vi "_Serial FPGA Send.vi"(0 "LED Control (T)":bool=TRUE) -> ()   [LabVIEW 2012]
uses:
  <vilib>/rvi/Emulation/niFpgaSctlEmulationGetInTimedLoop.vi
  <vilib>/rvi/Emulation/niFpgaSctlEmulationGlobalWrite.vi
  <vilib>/rvi/Memory/Memory_Emulation/nirvimemoryEmulationManagerCache_ReleaseExclusive.vi
  <vilib>/rvi/Memory/Memory_Emulation/niFpgaMemoryEmulationValidateCache.vi
  <vilib>/rvi/Memory/Memory_Emulation/nirvimemoryEmulationManagerCache_MakeExclusive.vi
  <vilib>/rvi/Memory/Memory_Emulation/niFpgaMemoryEmulationCacheClearOnFirstRun.vi
  <vilib>/rvi/DataTransferAndStorage/Container/Common/niFpgaContainerGetUniqueNameForEmu.vi
  <vilib>/rvi/Memory/Memory_Emulation/nirvimemoryEmulationManagerCache_InsertValue.vi
  <vilib>/Utility/error.llb/Clear Errors.vi
  <vilib>/rvi/Memory/Memory_Emulation/nirvimemoryEmulationManagerCache_SetValue.vi
  <vilib>/rvi/Memory/Memory_Emulation/nirvimemoryEmulationManagerCache_GetValue.vi
  <vilib>/rvi/Emulation/niFpgaSctlEmulationResourceMgr.vi
  <vilib>/rvi/eio/common/nirviEmuTemplateMethod_errors.vi
  <vilib>/rvi/DataTransferAndStorage/Container/XNode/niFpgaContainer.xnode
  <vilib>/rvi/Memory/Memory_Emulation/nirvimemoryEmulation.vi
  <vilib>/eio/EIONode/EIONode.xnode
  <vilib>/eio/EIOMethodNode/EIOMethodNode.xnode
panel:
  out "Bytes Written":u8
  out "Bytes Read":u8
  out "Done":bool
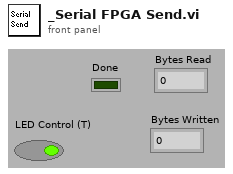
[diagram p1: front panel]
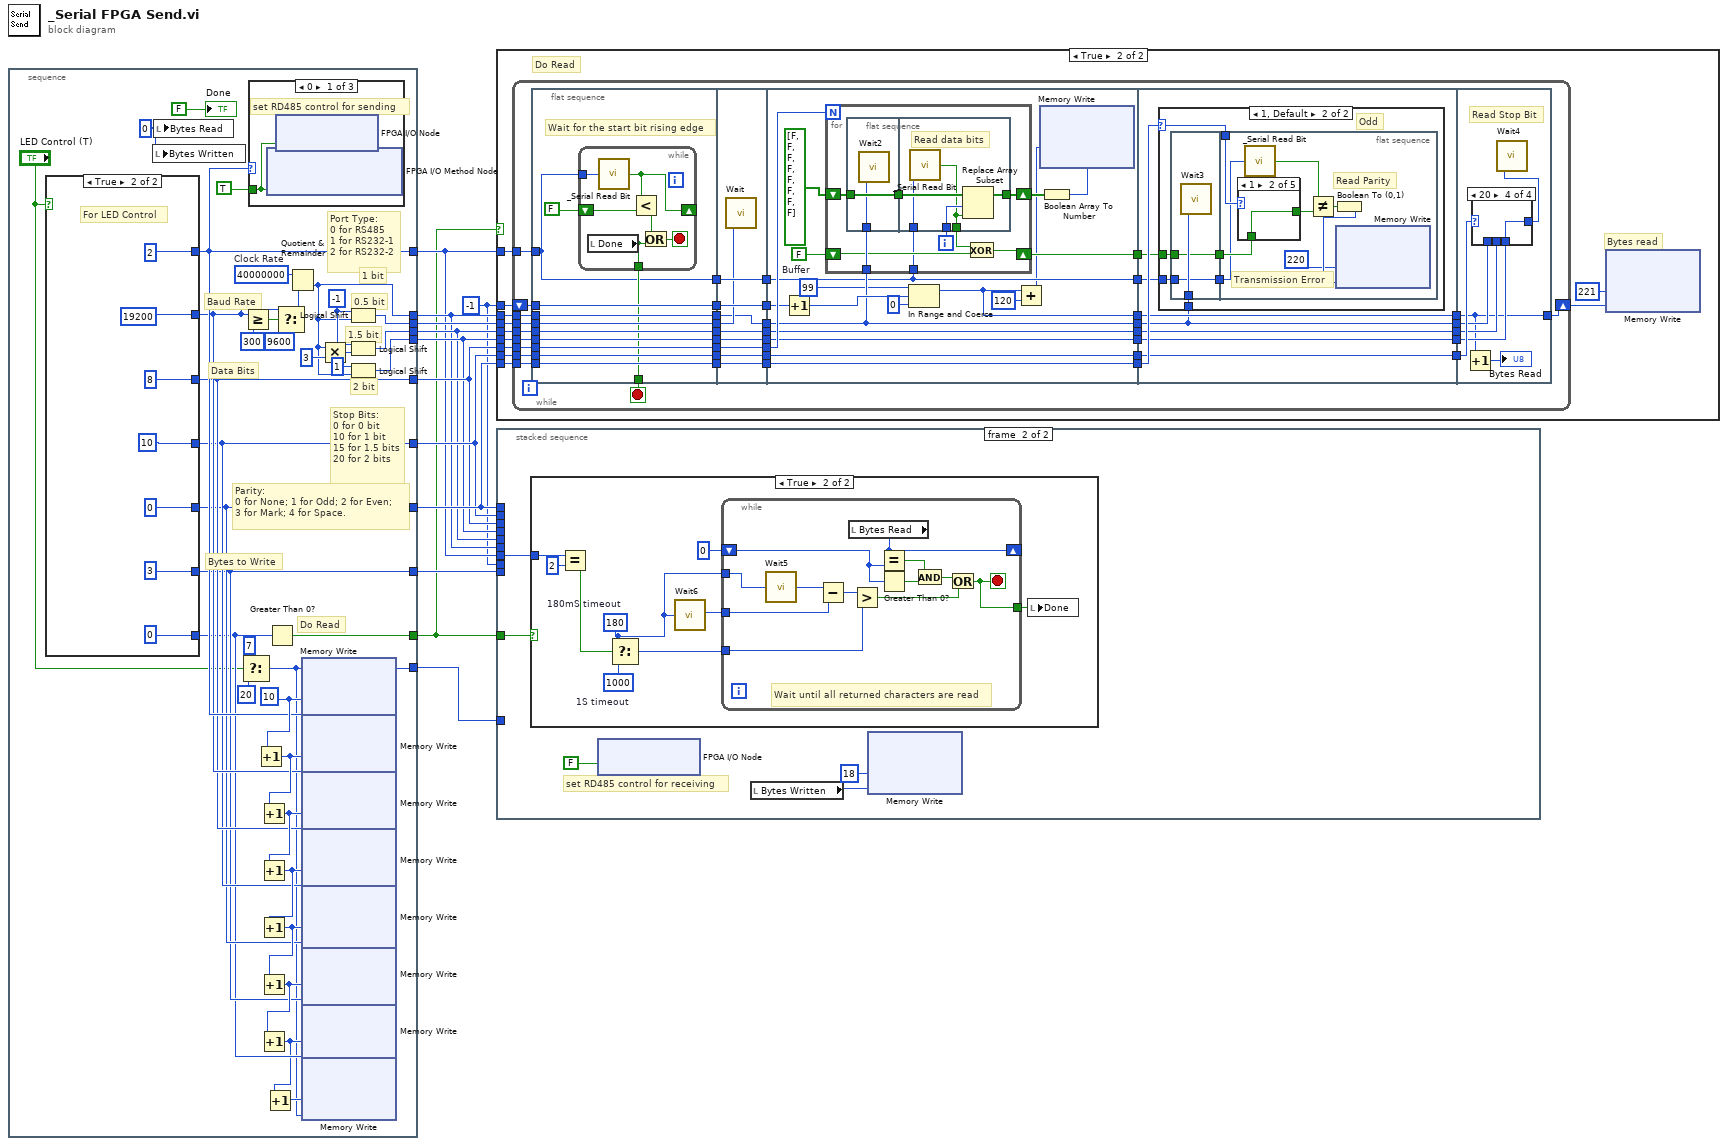
[diagram p0: block diagram]
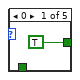
[diagram p4: hidden frame]
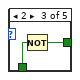
[diagram p5: hidden frame]
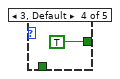
[diagram p6: hidden frame]
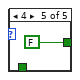
[diagram p7: hidden frame]
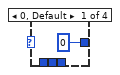
[diagram p8: hidden frame]
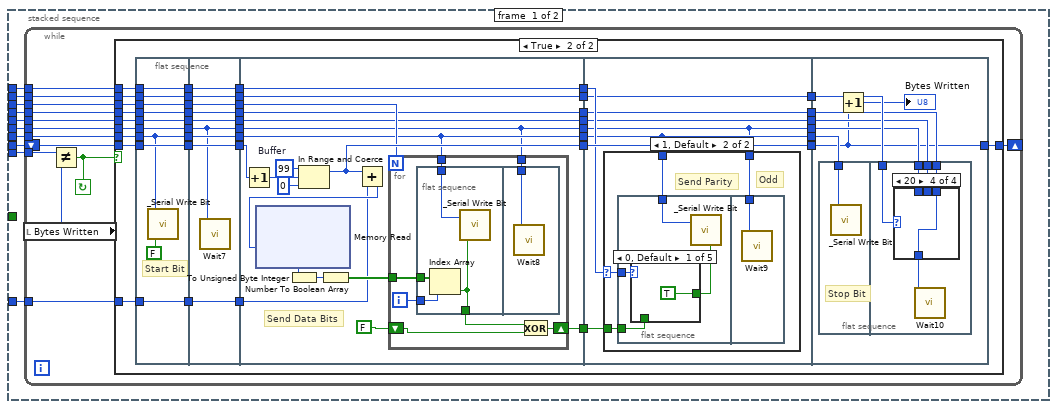
[diagram p11: hidden frame]
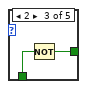
[diagram p15: hidden frame]
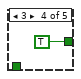
[diagram p16: hidden frame]
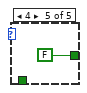
[diagram p17: hidden frame]
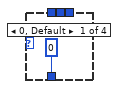
[diagram p18: hidden frame]
diagram:
  w3 = i16 -1
  n1 = stacked-sequence {
    tunnel: [w37] -> w5
    tunnel: [w40] -> w12
    tunnel: [w39] -> w6
    tunnel: [w36] -> w7
    tunnel: [w22] -> w8
    tunnel: [w24] -> w4
    tunnel: [w21] -> w9
    tunnel: [w20] -> w10
    tunnel: [w19] -> w11
    tunnel: [w32] -> w2
    tunnel: [w15] -> w1
    frame #0 {
      w29 = u8 10 ("Address")
      w42 = i16 -1 ("y")
      w44 = u32 40000000  # Clock Rate
      w34 = u8 0 ("Bytes Read")
      # "Do Read"
      # "1.5 bit"
      # "2 bit"
      # "0.5 bit"
      # "1 bit"
      # "Bytes to Write"
      # "Parity:\n0 for None; 1 for Odd; 2 for Even;\n3 for Mark; 4 for Space."
      # "Stop Bits:\n0 for 0 bit\n10 for 1 bit\n15 for 1.5 bits\n20 for 2 bits"
      # "Data Bits"
      # "Baud Rate"
      # "Port Type: \n0 for RS485\n1 for RS232-1\n2 for RS232-2"
      n2 = case shown="True" "LED Control (T)" {
        tunnel: [w57 u8 8 ("Address")] -> w22
        tunnel: [w56 u8 10 ("Address")] -> w21
        tunnel: [w55 u8 0 ("Address")] -> w20
        tunnel: [w54 u8 3 ("Address")] -> w19
        tunnel: [w53 u16 19200 ("Address")] -> w23
        tunnel: [w52 u8 2 ("Address")] -> w24
        tunnel: [w49 u8 0 ("Address")] -> w18
        frame False {
          w62 = u8 0 ("Address")
          n3 = Increment(x=w62) -> (x+1=w61:u8)
          n4 = Increment(x=w61) -> (x+1=w60:u8)
          n5 = Increment(x=w60) -> (x+1=w59:u8)
          n6 = Increment(x=w59) -> (x+1=w58:u8)
          n7 = Increment(x=w58) -> (x+1=w50:u8)
          n8 = Increment(x=w50) -> (x+1=w51:u8)
          n9 = xnode ("Memory Read")("Address"=w62) -> ("Data"=w52:u32)  [unwired: 1 in, 1 out]
          n10 = xnode ("Memory Read")("Address"=w61) -> ("Data"=w53:u32)  [unwired: 1 in, 1 out]
          n11 = xnode ("Memory Read")("Address"=w60) -> ("Data"=w57:u32)  [unwired: 1 in, 1 out]
          n12 = xnode ("Memory Read")("Address"=w59) -> ("Data"=w56:u32)  [unwired: 1 in, 1 out]
          n13 = xnode ("Memory Read")("Address"=w58) -> ("Data"=w55:u32)  [unwired: 1 in, 1 out]
          n14 = xnode ("Memory Read")("Address"=w50) -> ("Data"=w54:u32)  [unwired: 1 in, 1 out]
          n15 = xnode ("Memory Read")("Address"=w51) -> ("Data"=w49:u32)  [unwired: 1 in, 1 out]
        }
        frame True {
          # "For LED Control"
        }
      }
      n16 = local write "Bytes Written"(w34) -> ()
      n17 = local write "Bytes Read"(w34) -> ()
      n18 = Select(t=u8 7 ("y"), s="LED Control (T)", f=u8 20 ("y")) -> (s? t:f=w15:u8)
      n19 = Greater Or Equal?(x=w23, y=u16 300) -> (x >= y?=w47:bool)
      n20 = case shown="0" w24 {
        tunnel: TRUE -> [w70 w71 w72]
        frame 0 {
          # "set RD485 control for sending"
          n21 = xnode "FPGA I/O Method Node"("Enable"=w70) -> ()  [unwired: 1 in, 1 out]
          n22 = xnode "FPGA I/O Node"("Port5/DIO4"=w70) -> ()  [unwired: 1 in, 1 out]
        }
        frame 1, Default {
          n23 = xnode "FPGA I/O Method Node"("Enable"=w71) -> ()  [unwired: 1 in, 1 out]
        }
        frame 2 {
          # "LCD/LED Control"
          n24 = xnode "FPGA I/O Method Node"("Enable"=w72) -> ()  [unwired: 1 in, 1 out]
        }
      }
      n25 = Increment(x=w29) -> (x+1=w30:u8)
      n26 = Increment(x=w30) -> (x+1=w28:u8)
      n27 = Increment(x=w28) -> (x+1=w27:u8)
      n28 = Increment(x=w27) -> (x+1=w26:u8)
      n29 = Increment(x=w26) -> (x+1=w25:u8)
      n30 = Increment(x=w25) -> (x+1=w16:u8)
      n31 = Increment(x=w16) -> (x+1=w17:u8)
      n32 = Greater Than 0?(x=w18) -> (x > 0?=w32:bool)
      n33 = Select(t=w23, s=w47, f=u16 9600) -> (s? t:f=w45:u32)
      n34 = Quotient & Remainder(x=w44, y=w45) -> (floor(x/y)=w37:u32)  [unwired: 1 out]
      n35 = xnode ("Memory Write")("Address"=w29, "Data"=w24) -> ()  [unwired: 1 in, 1 out]
      n36 = xnode ("Memory Write")("Address"=w30, "Data"=w23) -> ()  [unwired: 1 in, 1 out]
      n37 = xnode ("Memory Write")("Address"=w28, "Data"=w22) -> ()  [unwired: 1 in, 1 out]
      n38 = xnode ("Memory Write")("Address"=w27, "Data"=w21) -> ()  [unwired: 1 in, 1 out]
      n39 = xnode ("Memory Write")("Address"=w26, "Data"=w20) -> ()  [unwired: 1 in, 1 out]
      n40 = xnode ("Memory Write")("Address"=w25, "Data"=w19) -> ()  [unwired: 1 in, 1 out]
      n41 = xnode ("Memory Write")("Address"=w16, "Data"=w18) -> ()  [unwired: 1 in, 1 out]
      n42 = xnode ("Memory Write")("Address"=w17, "Data"=w15) -> ()  [unwired: 1 in, 1 out]
      n43 = Multiply(x=w37, y=u32 3) -> (x*y=w41:u32)
      n44 = Logical Shift(y=w42, x=w37) -> (x << y=w40:u32)
      n45 = Logical Shift(y=w42, x=w41) -> (x << y=w39:u32)
      n46 = Logical Shift(y=i16 1, x=w37) -> (x << y=w36:u32)
      "Done" <- FALSE ("Done")
    }
  }
  n47 = case shown="True" w2 {
    tunnel: w12 -> [_ w83]
    tunnel: w10 -> [_ w82]
    tunnel: w9 -> [_ w81]
    tunnel: w8 -> [_ w80]
    tunnel: w7 -> [_ w79]
    tunnel: w6 -> [_ w78]
    tunnel: w5 -> [_ w77]
    tunnel: w4 -> [_ w76]
    tunnel: w3 -> [_ w75]
    frame False {
    }
    frame True {
      # "Bytes read"
      # "Do Read"
      n48 = while {
        tunnel: w79 -> [w121]
        tunnel: w78 -> [w122]
        tunnel: w83 -> [w123]
        tunnel: w77 -> [w124]
        tunnel: w76 -> [w104]
        shift-right: [w84] -> w73
        shift-left: w75 -> [w102]
        tunnel: w80 -> [w120]
        tunnel: w81 -> [w119]
        tunnel: w82 -> [w118]
        stop <- w85 stop-if-true
        n49 = flat-sequence {
          tunnel: w118 -> [w129]
          tunnel: w119 -> [w130]
          tunnel: w120 -> [w131]
          tunnel: w121 -> [w132]
          tunnel: w122 -> [w133]
          tunnel: w123 -> [w134]
          tunnel: w124 -> [w135]
          tunnel: [w135] -> w111
          tunnel: [w134] -> w110
          tunnel: [w133] -> w109
          tunnel: [w132] -> w108
          tunnel: [w131] -> w107
          tunnel: [w130] -> w106
          tunnel: [w129] -> w105
          tunnel: w104 -> [w125]
          tunnel: [w128] -> w103
          tunnel: w102 -> [w128]
          tunnel: [w125] -> w99
          tunnel: [w126] -> w85
          tunnel: [w142] -> w117
          tunnel: [w150] -> w116
          tunnel: [w149] -> w115
          tunnel: [w148] -> w114
          tunnel: [w147] -> w113
          tunnel: [w146] -> w112
          tunnel: w111 -> [w142]
          tunnel: w110 -> [w143]
          tunnel: w109 -> [w150]
          tunnel: w108 -> [w149]
          tunnel: w107 -> [w148]
          tunnel: w106 -> [w147]
          tunnel: w105 -> [w146]
          tunnel: w103 -> [w145]
          tunnel: [w145] -> w101
          tunnel: [w144] -> w100
          tunnel: w99 -> [w144]
          tunnel: w117 -> [w159]
          tunnel: w116 -> [w156]
          tunnel: w115 -> [w155]
          tunnel: w114 -> [w167]
          tunnel: w113 -> [w157]
          tunnel: w112 -> [w160]
          tunnel: w101 -> [w166]
          tunnel: w100 -> [w154]
          tunnel: [w161] -> w98
          tunnel: [w160] -> w97
          tunnel: [w159] -> w96
          tunnel: [w154] -> w95
          tunnel: [w158] -> w94
          tunnel: [w157] -> w91
          tunnel: [w156] -> w88
          tunnel: [w155] -> w86
          tunnel: w98 -> [w192]
          tunnel: w97 -> [w193]
          tunnel: w96 -> [w188]
          tunnel: w95 -> [w191]
          tunnel: w94 -> [w190]
          tunnel: [w190] -> w93
          tunnel: [w189] -> w92
          tunnel: w91 -> [w189]
          tunnel: [w188] -> w90
          tunnel: [w187] -> w89
          tunnel: w88 -> [w187]
          tunnel: [w186] -> w87
          tunnel: w86 -> [w186]
          tunnel: w93 -> [w218]
          tunnel: w92 -> [w223]
          tunnel: w90 -> [w221]
          tunnel: w89 -> [w220]
          tunnel: w87 -> [w219]
          tunnel: [w218] -> w84
          frame #0 {
            # "Wait for the start bit rising edge"
            n50 = while {
              shift-right: [w137] -> _
              shift-left: FALSE -> [w141]
              tunnel: w125 -> [w140]
              tunnel: [w136] -> w126
              stop <- w138 stop-if-true
              n51 = local read "Done"() -> (w136:bool)
              n52 = call "_Serial Read Bit.vi"("Port type"=w140) -> ("BitState"=w137:bool)
              n53 = Less?(x=w137, y=w141) -> (x < y?=w139:bool)
              n54 = Or(x=w139, y=w136) -> (x .or. y?=w138:bool)
            }
          }
          frame #1 {
            n55 = call "Wait"("Count(Ticks)"=w143) -> ()  [unwired: 1 out]
          }
          frame #2 {
            w152 = i16 99  # Buffer
            n56 = Increment(x=w166) -> (x+1=w165:i16)
            n57 = for {
              N: w167 -> [_]
              shift-right: [w172] -> w162
              shift-left: bool[] [FALSE, FALSE, FALSE, FALSE, FALSE, FALSE, FALSE, FALSE] -> [w178]
              tunnel: w159 -> [w176]
              shift-right: [w175] -> w161
              shift-left: FALSE -> [w174]
              tunnel: w154 -> [w170]
              i -> [w171]
              n58 = flat-sequence {
                tunnel: w178 -> [w180]
                tunnel: [w180] -> w177
                tunnel: w176 -> [w179]
                tunnel: w171 -> [w185]
                tunnel: w177 -> [w184]
                tunnel: [w183] -> w172
                tunnel: [w181] -> w173
                tunnel: w170 -> [w182]
                frame #0 {
                  n59 = call "Wait2"("Count(Ticks)"=w179) -> ()  [unwired: 1 out]
                }
                frame #1 {
                  # "Read data bits"
                  n60 = call "_Serial Read Bit.vi"("Port type"=w182) -> ("BitState"=w181:bool)
                  n61 = Replace Array Subset(array=w184, new element=w181, index=w185) -> (w183:bool[])
                }
              }
              n62 = Exclusive Or(1:w174, 2:w173) -> (0:w175:bool)
            }
            n63 = In Range and Coerce(upper limit=w152, x=w165, lower limit=i16 0) -> (coerced(x)=w158:i16)  [unwired: 1 out]
            n64 = Add(x=w158, y=i16 120) -> (x+y=w153:i16)
            n65 = Boolean Array To Number(Boolean array=w162) -> (number=w151:u8)
            n66 = xnode ("Memory Write")("Address"=w153, "Data"=w151) -> ()  [unwired: 1 in, 1 out]
          }
          frame #3 {
            n67 = case shown="1, Default" w193 {
              selector: w193 -> [_ w198]
              tunnel: w192 -> [_ w196]
              tunnel: w188 -> [_ w199]
              tunnel: w191 -> [_ w194]
              frame 0 {
                # "None"
              }
              frame 1, Default {
                # "Odd"
                n68 = flat-sequence {
                  tunnel: w199 -> [w202]
                  tunnel: [w201] -> w197
                  tunnel: w196 -> [w201]
                  tunnel: [w200] -> w195
                  tunnel: w194 -> [w200]
                  tunnel: w198 -> [w210]
                  tunnel: w197 -> [w208]
                  tunnel: w195 -> [w204]
                  frame #0 {
                    n69 = call "Wait3"("Count(Ticks)"=w202) -> ()  [unwired: 1 out]
                  }
                  frame #1 {
                    # "Read Parity"
                    # "Transmission Error"
                    n70 = case shown="1" w210 {
                      tunnel: w208 -> [_ w212 w214 _ _]
                      tunnel: [TRUE ("y") w212 w213 TRUE ("y") FALSE ("y")] -> w209
                      frame 0 {
                      }
                      frame 1 {
                      }
                      frame 2 {
                        n71 = Not(x=w214) -> (.not. x?=w213:bool)
                      }
                      frame 3, Default {
                      }
                      frame 4 {
                      }
                    }
                    n72 = call "_Serial Read Bit.vi"("Port type"=w204) -> ("BitState"=w203:bool)
                    n73 = Not Equal?(x=w203, y=w209) -> (x != y?=w207:bool)
                    n74 = Boolean To (0,1)(Boolean=w207) -> (0, 1=w206:i16)
                    n75 = xnode ("Memory Write")("Address"=u16 220 ("y"), "Data"=w206) -> ()  [unwired: 1 in, 1 out]
                  }
                }
              }
            }
          }
          frame #4 {
            # "Read Stop Bit"
            n76 = Increment(x=w218) -> (x+1=→"Bytes Read":i16)
            n77 = case shown="20" w223 {
              tunnel: w221 -> [_ w225 _ _]
              tunnel: w220 -> [_ _ w226 _]
              tunnel: w219 -> [_ _ _ w227]
              tunnel: [u32 0 ("One Bit") w225 w226 w227] -> w222
              frame 0, Default {
              }
              frame 10 {
              }
              frame 15 {
              }
              frame 20 {
              }
            }
            n78 = call "Wait4"("Count(Ticks)"=w222) -> ()  [unwired: 1 out]
          }
        }
      }
      n79 = xnode ("Memory Write")("Address"=u16 221 ("y"), "Data"=w73) -> ()  [unwired: 1 in, 1 out]
    }
  }
  n80 = stacked-sequence {
    tunnel: w11 -> [w237 _]
    tunnel: w10 -> [w236 _]
    tunnel: w9 -> [w235 _]
    tunnel: w8 -> [w234 _]
    tunnel: w7 -> [w233 _]
    tunnel: w6 -> [w232 _]
    tunnel: w5 -> [w231 _]
    tunnel: w4 -> [w230 w384]
    tunnel: w3 -> [w229 _]
    tunnel: w2 -> [_ w387]
    tunnel: w1 -> [w228 _]
    frame #0 {
      n81 = while {
        tunnel: w237 -> [w250]
        tunnel: w236 -> [w247]
        tunnel: w235 -> [w246]
        tunnel: w234 -> [w245]
        tunnel: w233 -> [w244]
        tunnel: w232 -> [w243]
        tunnel: w231 -> [w242]
        tunnel: w230 -> [w241]
        shift-right: [w239] -> _
        shift-left: w229 -> [w240]
        tunnel: w228 -> [w238]
        stop <- w248 continue-if-true
        n82 = local read "Bytes Written"() -> (w249:u8)
        n83 = Not Equal?(x=w250, y=w249) -> (x != y?=w248:bool)
        n84 = case shown="True" w248 {
          tunnel: w247 -> [_ w275]
          tunnel: w246 -> [_ w266]
          tunnel: w245 -> [_ w284]
          tunnel: w244 -> [_ w255]
          tunnel: w243 -> [_ w260]
          tunnel: w242 -> [_ w289]
          tunnel: w241 -> [_ w293]
          tunnel: w240 -> [w251 w291]
          tunnel: [w251 w287] -> w239
          tunnel: w238 -> [_ w252]
          frame False {
          }
          frame True {
            n85 = flat-sequence {
              tunnel: w293 -> [w300]
              tunnel: [w303] -> w292
              tunnel: w291 -> [w303]
              tunnel: [w302] -> w290
              tunnel: w289 -> [w302]
              tunnel: [w301] -> w285
              tunnel: w284 -> [w301]
              tunnel: [w300] -> w282
              tunnel: [w299] -> w276
              tunnel: w275 -> [w299]
              tunnel: [w298] -> w267
              tunnel: w266 -> [w298]
              tunnel: [w297] -> w261
              tunnel: w260 -> [w297]
              tunnel: [w296] -> w256
              tunnel: w255 -> [w296]
              tunnel: [w294] -> w253
              tunnel: w252 -> [w294]
              tunnel: w292 -> [w312]
              tunnel: w290 -> [w309]
              tunnel: [w312] -> w288
              tunnel: [w311] -> w286
              tunnel: w285 -> [w311]
              tunnel: [w310] -> w283
              tunnel: w282 -> [w310]
              tunnel: [w309] -> w281
              tunnel: [w308] -> w277
              tunnel: w276 -> [w308]
              tunnel: [w307] -> w268
              tunnel: w267 -> [w307]
              tunnel: [w306] -> w262
              tunnel: w261 -> [w306]
              tunnel: [w305] -> w257
              tunnel: w256 -> [w305]
              tunnel: [w304] -> w254
              tunnel: w253 -> [w304]
              tunnel: w288 -> [w331]
              tunnel: w286 -> [w323]
              tunnel: w283 -> [w318]
              tunnel: w281 -> [w317]
              tunnel: [w324] -> w280
              tunnel: [w320] -> w279
              tunnel: [w319] -> w278
              tunnel: w277 -> [w319]
              tunnel: [w318] -> w274
              tunnel: [w317] -> w273
              tunnel: [w316] -> w269
              tunnel: w268 -> [w316]
              tunnel: [w315] -> w263
              tunnel: w262 -> [w315]
              tunnel: [w314] -> w258
              tunnel: w257 -> [w314]
              tunnel: w254 -> [w313]
              tunnel: w280 -> [w351]
              tunnel: w279 -> [w349]
              tunnel: w278 -> [w350]
              tunnel: w274 -> [w348]
              tunnel: w273 -> [w346]
              tunnel: [w351] -> w272
              tunnel: [w348] -> w271
              tunnel: [w347] -> w270
              tunnel: w269 -> [w347]
              tunnel: [w346] -> w265
              tunnel: [w345] -> w264
              tunnel: w263 -> [w345]
              tunnel: [w344] -> w259
              tunnel: w258 -> [w344]
              tunnel: [w368] -> w287
              tunnel: w272 -> [w368]
              tunnel: w271 -> [w373]
              tunnel: w270 -> [w372]
              tunnel: w265 -> [w371]
              tunnel: w264 -> [w370]
              tunnel: w259 -> [w369]
              frame #0 {
                # "Start Bit"
                n86 = call "_Serial Write Bit.vi"("BitState(T)"=FALSE, "Port type"=w300) -> ()  [unwired: 1 out]
              }
              frame #1 {
                n87 = call "Wait7"("Count(Ticks)"=w309) -> ()  [unwired: 1 out]
              }
              frame #2 {
                w329 = i16 99  # Buffer
                # "Send Data Bits"
                n88 = Increment(x=w331) -> (x+1=w330:i16)
                n89 = In Range and Coerce(upper limit=w329, x=w330, lower limit=i16 0) -> (coerced(x)=w324:i16)  [unwired: 1 out]
                n90 = Add(x=w324, y=w313) -> (x+y=w327:i16)
                n91 = xnode ("Memory Read")("Address"=w327) -> ("Data"=w325:u32)  [unwired: 1 in, 1 out]
                n92 = To Unsigned Byte Integer(number=w325) -> (unsigned 8bit integer=w326:u8)
                n93 = Number To Boolean Array(number=w326) -> (Boolean array=w322:bool[])
                n94 = for {
                  N: w323 -> [_]
                  tunnel: w322 -> [w338]
                  shift-right: [w336] -> w320
                  shift-left: FALSE -> [w335]
                  tunnel: w318 -> [w333]
                  tunnel: w317 -> [w332]
                  i -> [w337]
                  n95 = flat-sequence {
                    tunnel: w338 -> [w342]
                    tunnel: w337 -> [w341]
                    tunnel: [w339] -> w334
                    tunnel: w333 -> [w340]
                    tunnel: w332 -> [w343]
                    frame #0 {
                      n96 = Index Array(array=w342, index=w341) -> (element=w339:bool)
                      n97 = call "_Serial Write Bit.vi"("BitState(T)"=w339, "Port type"=w340) -> ()  [unwired: 1 out]
                    }
                    frame #1 {
                      n98 = call "Wait8"("Count(Ticks)"=w343) -> ()  [unwired: 1 out]
                    }
                  }
                  n99 = Exclusive Or(1:w335, 2:w334) -> (0:w336:bool)
                }
              }
              frame #3 {
                n100 = case shown="1, Default" w350 {
                  selector: w350 -> [_ w355]
                  tunnel: w349 -> [_ w354]
                  tunnel: w348 -> [_ w353]
                  tunnel: w346 -> [_ w352]
                  frame 0 {
                    # "None"
                  }
                  frame 1, Default {
                    # "Send Parity"
                    # "Odd"
                    n101 = flat-sequence {
                      tunnel: w355 -> [w359]
                      tunnel: w354 -> [w358]
                      tunnel: w353 -> [w356]
                      tunnel: w352 -> [w366]
                      frame #0 {
                        n102 = case shown="0, Default" w359 {
                          tunnel: w358 -> [_ w361 w363 _ _]
                          tunnel: [TRUE ("y") w361 w362 TRUE ("y") FALSE ("y")] -> w357
                          frame 0, Default {
                          }
                          frame 1 {
                          }
                          frame 2 {
                            n103 = Not(x=w363) -> (.not. x?=w362:bool)
                          }
                          frame 3 {
                          }
                          frame 4 {
                          }
                        }
                        n104 = call "_Serial Write Bit.vi"("BitState(T)"=w357, "Port type"=w356) -> ()  [unwired: 1 out]
                      }
                      frame #1 {
                        n105 = call "Wait9"("Count(Ticks)"=w366) -> ()  [unwired: 1 out]
                      }
                    }
                  }
                }
              }
              frame #4 {
                n106 = flat-sequence {
                  tunnel: w373 -> [w374]
                  tunnel: w372 -> [w379]
                  tunnel: w371 -> [w377]
                  tunnel: w370 -> [w376]
                  tunnel: w369 -> [w375]
                  frame #0 {
                    # "Stop Bit"
                    n107 = call "_Serial Write Bit.vi"("Port type"=w374) -> ()  [unwired: 1 in, 1 out]
                  }
                  frame #1 {
                    n108 = case shown="20" w379 {
                      tunnel: [u32 0 ("One Bit") w381 w382 w383] -> w378
                      tunnel: w377 -> [_ w381 _ _]
                      tunnel: w376 -> [_ _ w382 _]
                      tunnel: w375 -> [_ _ _ w383]
                      frame 0, Default {
                      }
                      frame 10 {
                      }
                      frame 15 {
                      }
                      frame 20 {
                      }
                    }
                    n109 = call "Wait10"("Count(Ticks)"=w378) -> ()  [unwired: 1 out]
                  }
                }
                n110 = Increment(x=w368) -> (x+1=→"Bytes Written":i16)
              }
            }
          }
        }
      }
    }
    frame #1 {
      # "set RD485 control for receiving"
      n111 = case shown="True" w387 {
        tunnel: w384 -> [_ w394]
        frame False {
        }
        frame True {
          w389 = u32 180  # 180mS timeout
          w391 = u32 1000  # 1S timeout
          n112 = Equal?(x=w394, y=u32 2) -> (x = y?=w392:bool)
          n113 = Select(t=w389, s=w392, f=w391) -> (s? t:f=w390:u32)
          n114 = call "Wait6"("Count(mSec)"=w389) -> ("Tick Count(mSec)"=w395:u32)
          n115 = while {
            tunnel: w395 -> [w408]
            shift-right: [w406] -> _
            shift-left: u8 0 ("Bytes Read") -> [w405]
            tunnel: [w400] -> w396
            tunnel: w389 -> [w399]
            tunnel: w390 -> [w398]
            stop <- w400 stop-if-true
            # "Wait until all returned characters are read"
            n116 = call "Wait5"("Count(mSec)"=w399) -> ("Tick Count(mSec)"=w409:u32)
            n117 = Subtract(x=w409, y=w408) -> (x-y=w407:u32)
            n118 = local read "Bytes Read"() -> (w406:u8)
            n119 = Greater?(x=w407, y=w398) -> (0:w401:bool)
            n120 = Equal?(x=w406, y=w405) -> (x = y?=w403:bool)
            n121 = Greater Than 0?(x=w405) -> (x > 0?=w404:bool)
            n122 = And(x=w403, y=w404) -> (x .and. y?=w402:bool)
            n123 = Or(x=w402, y=w401) -> (x .or. y?=w400:bool)
          }
          n124 = local write "Done"(w396) -> ()
        }
      }
      n125 = xnode "FPGA I/O Node"("Port5/DIO4"=FALSE) -> ()  [unwired: 1 in, 1 out]
      n126 = local read "Bytes Written"() -> (w386:u8)
      n127 = xnode ("Memory Write")("Address"=u8 18, "Data"=w386) -> ()  [unwired: 1 in, 1 out]
    }
  }
